vi "Upd Flow Measured.vi"(8 "error in (no error)":errorcluster, 10 "MFC Percent":T1, 11 "C100L in":refnum<class "C100L.lvclass">) -> (0 "error out":errorcluster, 3 "C100L out":refnum<class "C100L.lvclass">)   [LabVIEW 2021]
uses:
  <vilib>/addons/control/pid/NI_PID_pid.lvlib
  <vilib>/addons/control/pid/pid.llb/PID Percentage to EGU (DBL).vi
  C100L.lvclass
  C:/Program Files/National Instruments/LabVIEW 2021/vi.lib/MGI/Panel Manager/Panel Actor/Panel Actor/Panel Actor.lvclass
  C:/Program Files/National Instruments/LabVIEW 2021/vi.lib/ActorFramework/Actor/Actor.lvclass
  C:/PPLs/C100L/C100L/C100L.lvclass
  C:/PPLs/DAQ-arch/DAQ/AI Interface/AI Interface/AI Interface.lvclass
  MFC Percent.ctl
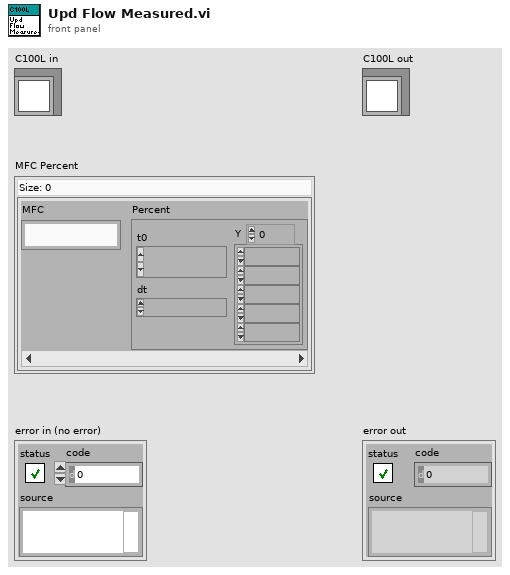
[diagram p1: front panel]
types:
  T1 = typedef "C100L.lvlib/C100L.lvclass/MFC Percent.ctl" = map{string, waveform(dbl)}
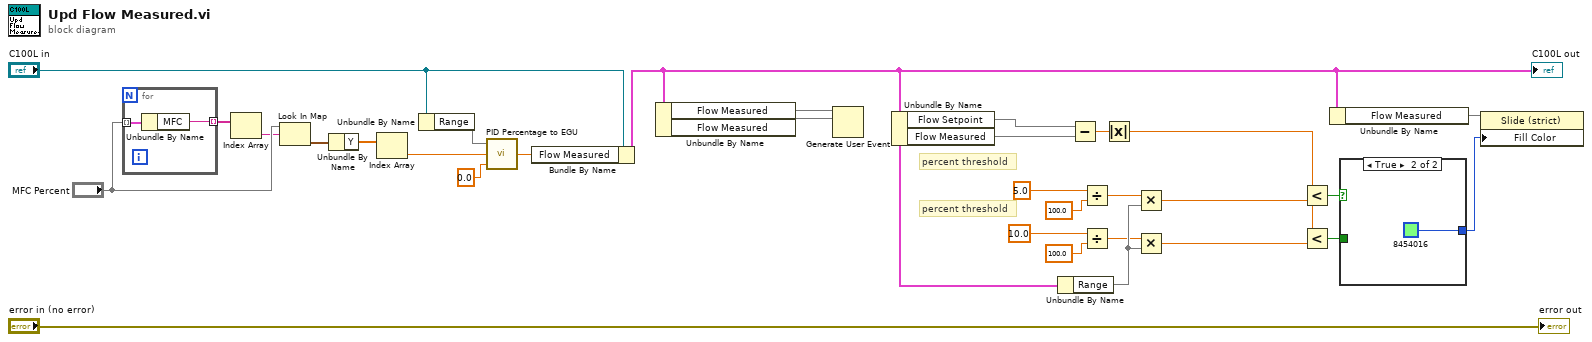
[diagram p0: block diagram]
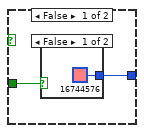
[diagram p2: hidden frame]
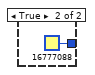
[diagram p3: hidden frame]
diagram:
  # "percent threshold"
  # "percent threshold"
  n1 = for {
    tunnel: "MFC Percent" -> [w33] mode=indexing
    tunnel: [w32] -> w3 mode=indexing
    n2 = Unbundle By Name(w33) -> ("MFC"=w32:string)
  }
  n3 = Index Array(array=w3) -> (element=w2:string)  [unwired: 1 in]
  n4 = Look In Map(map="MFC Percent", key=w2) -> (value=w1:waveform(dbl))  [unwired: 1 in, 1 out]
  n5 = Unbundle By Name(w1) -> ("Y"=w10:dbl[])
  n6 = Index Array(array=w10) -> (element=w9:dbl)  [unwired: 1 in]
  n7 = Unbundle By Name("C100L in") -> ("Range"=w5)
  n8 = call-poly <vilib>:"PID Percentage to EGU.vi"("minimum (EGU)"=0.0, "% span"=w9, "maximum (EGU)"=w5) -> ("output (EGU)"=w7:dbl)  [unwired: 1 in]
  n9 = Bundle By Name(cluster="C100L in", "Flow Measured"=w7) -> (w11:cluster{})
  "C100L out" <- w11
  n10 = Unbundle By Name(w11) -> ("Flow Measured"=w13, "Flow Measured"=w12)
  n11 = Generate User Event(user event=w13, event data cluster=w12) -> ()  [unwired: 2 in, 2 out]
  n12 = Unbundle By Name(w11) -> ("Flow Setpoint"=w27, "Flow Measured"=w20)
  n13 = Unbundle By Name(w11) -> ("Range"=w21)
  n14 = Subtract(x=w27, y=w20) -> (x-y=w28:dbl)
  n15 = Divide(x=5.0, y=100.0) -> (x/y=w14:dbl)
  n16 = Divide(x=10.0, y=100.0) -> (x/y=w19:dbl)
  n17 = Absolute Value(x=w28) -> (abs(x)=w24:dbl)
  n18 = Multiply(x=w14, y=w21) -> (x*y=w26:dbl)
  n19 = Multiply(x=w19, y=w21) -> (x*y=w25:dbl)
  n20 = Less?(x=w24, y=w26) -> (x < y?=w30:bool)
  n21 = Less?(x=w24, y=w25) -> (x < y?=w23:bool)
  n22 = Unbundle By Name(w11) -> ("Flow Measured"=w22)
  n23 = case shown="True" w30 {
    tunnel: [w34 u32 8454016 ("Fill Color")] -> w29
    tunnel: w23 -> [w35 _]
    frame False {
      n24 = case shown="False" w35 {
        tunnel: [u32 16744576 ("Fill Color") u32 16777088 ("Fill Color")] -> w34
        frame False {
        }
        frame True {
        }
      }
    }
    frame True {
    }
  }
  n25 = property class="Slide (strict)"(reference=w22, "Fill Color"=w29) -> ()  [unwired: 1 in, 2 out]
  "error out" <- "error in (no error)"
